vi "Amira Bladder Calibration.vi"() -> ()   [LabVIEW 2020]
uses:
  <userlib>/KQD LabVIEW User/Serial/Controls/SERIAL PortConfig.ctl
  <userlib>/KQD LabVIEW User/Serial/Controls/SERIAL BaudRate.ctl
  <userlib>/Amira UART/Public/TypeDefs/AUART StepDir.ctl
  <userlib>/Amira UART/Amira UART.lvclass
  <userlib>/KQD LabVIEW User/Serial/Serial.lvlib
panel:
  in  "RunWith":cluster{"Steps":i32, "Rates":i32}={"Steps"=400, "Rates"=40}
  in  "Folder":path=path "C:/Amira Data/Strip"
  in  "Strip":enum16{"Surface", "Blader"}(ring)
  out "FrontOpen":dbl
  out "BackOpen":dbl
  out "FrontClose":dbl
  out "BackClose":dbl
  in  "StartAt":cluster{"Steps":i32, "Rates":i32}={"Steps"=950, "Rates"=200}
  out "Position":dbl[](graph)
  in  "DAQ":tag="Dev1/port0"
  out "UART":string
  in  "ComPort":refnum<visa-resource-name>
  in  "Config":T1={"BaudRate"=enum."460800", "StopBits"=10, "DataBits"=8, "Parity"=enum."None", "FlowControl"=2, "TimeOut"=1000, "TermChar"=10, "ReadTermEn"=TRUE} {"TermChar" format="%.0x"; "FlowControl" items=["None", "XON/XOFF", "RTS/CTS", "XON/XOFF & RTS/CTS", "DTR/DSR", "XON/XOFF & DTR/DSR"]; "DataBits" min=5 max=8 step=1; "StopBits" items=["1.0"=10, "1.5"=15, "2.0"=20]}
  out "ErrOut":errorcluster
  in  "ErrIn":errorcluster
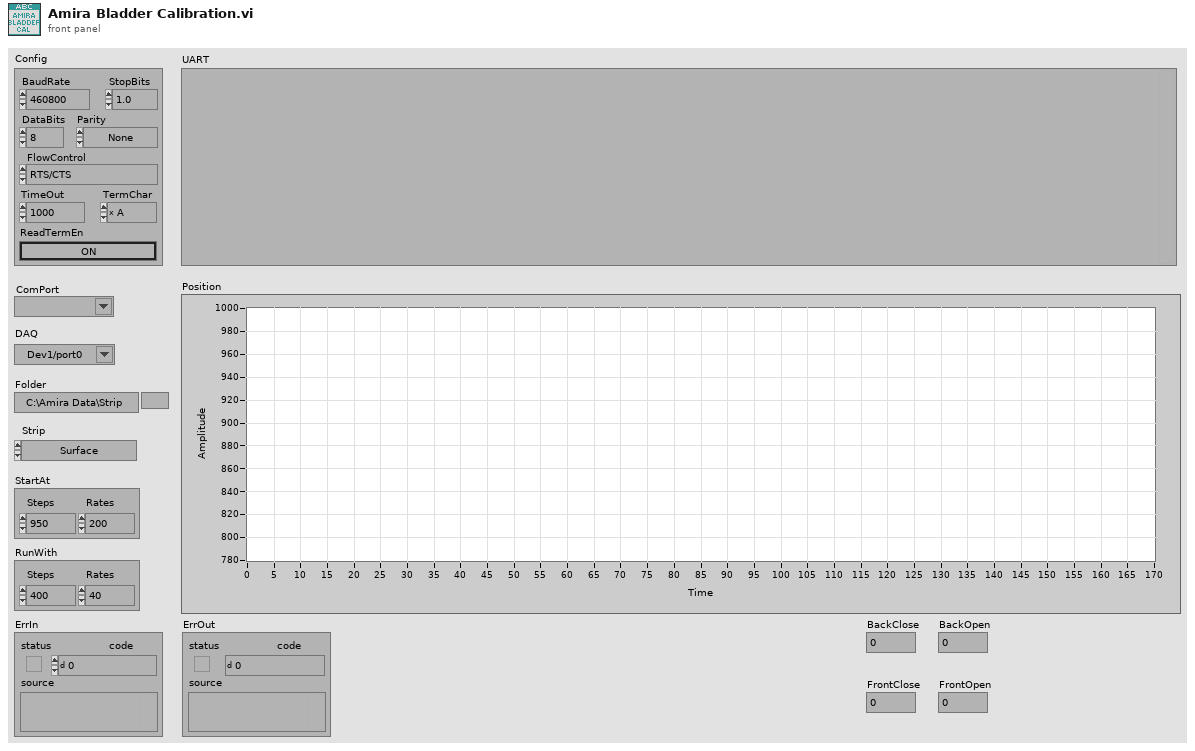
[diagram p1: front panel]
types:
  T1 = typedef "Serial.lvlib/SERIAL PortConfig.ctl" = cluster{"BaudRate":T2, "StopBits":u16, "DataBits":u16, "Parity":enum16{"None", "Odd", "Even", "Mark", "Space"}, "FlowControl":u16, "TimeOut":u32, "TermChar":u8, "ReadTermEn":bool}
  T2 = typedef "SERIAL BaudRate.ctl" = enum16{"2400", "4800", "7200", "9600", "14400", "19200", "28800", "38400", "57600", "115200", "128000", "230400", "460800", "921600"}
  T3 = typedef "Amira UART.lvclass/AUART StepDir.ctl" = enum16{"", "compress", "decompress"}
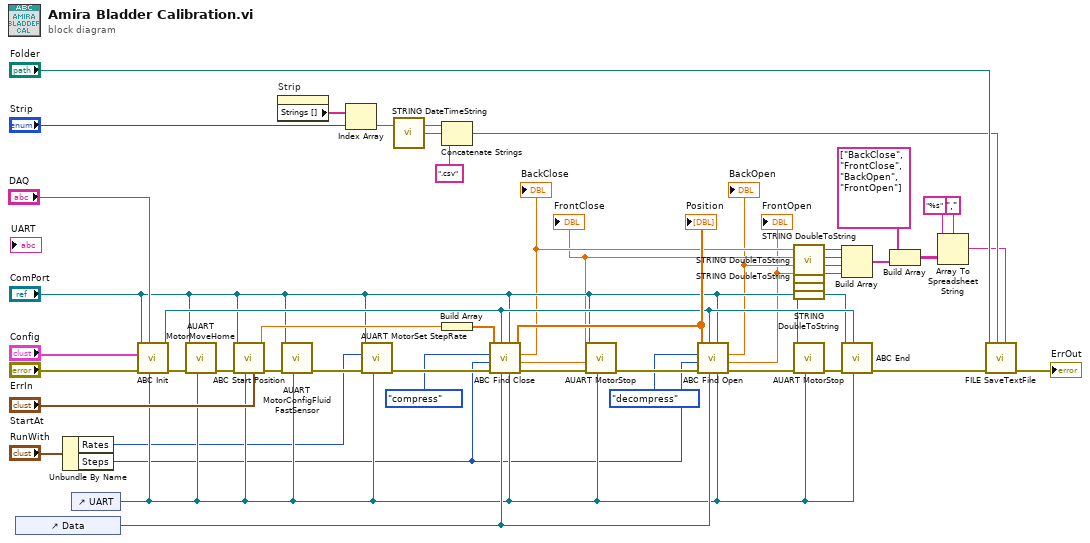
[diagram p0: block diagram]
diagram:
  n1 = control-ref of="Data"() -> (w32:refnum<vi>)
  n2 = Unbundle By Name("RunWith") -> ("Rates"=w2:i32, "Steps"=w1:i32)
  n3 = control-ref of="UART"() -> (w29:refnum<vi>)
  n4 = call "ABC Init.vi"("UART"=w29, "DAQ"="DAQ", "ErrIn"="ErrIn", "PortConfig"="Config", "ComPort"="ComPort") -> ("ErrOut"=w44:errorcluster, "DaqTask"=w33:refnum<k21>)  [unwired: 5 in]
  n5 = call <userlib>:"AUART MotorMoveHome.vi"("UART"=w29, "ErrIn"=w44, "Port"="ComPort") -> ("ErrOut"=w43:errorcluster)  [unwired: 7 in, 1 out]
  n6 = call "ABC Start Position.vi"("Start"="StartAt", "UART"=w29, "ErrIn"=w43, "ComPort"="ComPort") -> ("ErrOut"=w42:errorcluster, "LastPos"=w39:dbl)  [unwired: 6 in]
  n7 = property on="Strip" class="Enum (strict)"() -> ("Strings []"=w22:string[])  [unwired: 2 in, 2 out]
  n8 = call <userlib>:"AUART MotorConfigFluidFastSensor.vi"("UART"=w29, "ErrIn"=w42, "Port"="ComPort") -> ("ErrOut"=w46:errorcluster)  [unwired: 8 in]
  n9 = Index Array(array=w22, index="Strip") -> (element=w20:string)
  n10 = call <userlib>:"AUART MotorSet StepRate.vi"("UART"=w29, "ErrIn"=w46, "step_rate"=w2, "Port"="ComPort") -> ("ErrOut"=w45:errorcluster)  [unwired: 7 in]
  n11 = call <userlib>:"STRING DateTimeString.vi"() -> ("DateTimeStr"=w19:string)  [unwired: 2 in]
  n12 = Concatenate Strings(w20, w19, ".csv" ("string")) -> (w16:string)
  n13 = Build Array(w39) -> (w40:dbl[])
  n14 = call "ABC Find Close.vi"("UART"=w29, "ComPort"="ComPort", "Data"=w32, "DaqTask"=w33, "ErrIn"=w45, "#Step"=w1, "Dir"=AUART_StepDir."compress" ("step_dir"), "DataIn"=w40) -> ("ErrOut"=w37:errorcluster, "FrontClose"=w27:dbl, "BackClose"=w28:dbl, "DataOut"=w34:dbl[])
  "Position" <- w34
  "BackClose" <- w28
  "FrontClose" <- w27
  n15 = call <userlib>:"AUART MotorStop.vi"("UART"=w29, "ErrIn"=w37, "Port"="ComPort") -> ("ErrOut"=w36:errorcluster)  [unwired: 8 in]
  n16 = call "ABC Find Open.vi"("UART"=w29, "ComPort"="ComPort", "Data"=w32, "DaqTask"=w33, "ErrIn"=w36, "#Step"=w1, "Dir"=AUART_StepDir."decompress" ("step_dir"), "DataIn"=w34) -> ("ErrOut"=w35:errorcluster, "FrontOpen"=w25:dbl, "BackOpen"=w26:dbl)  [unwired: 1 out]
  "BackOpen" <- w26
  "FrontOpen" <- w25
  n17 = call <userlib>:"STRING DoubleToString.vi"("Num"=w28) -> ("DblStr"=w15:string)  [unwired: 3 in]
  n18 = call <userlib>:"STRING DoubleToString.vi"("Num"=w27) -> ("DblStr"=w14:string)  [unwired: 3 in]
  n19 = call <userlib>:"STRING DoubleToString.vi"("Num"=w26) -> ("DblStr"=w13:string)  [unwired: 3 in]
  n20 = call <userlib>:"STRING DoubleToString.vi"("Num"=w25) -> ("DblStr"=w12:string)  [unwired: 3 in]
  n21 = call <userlib>:"AUART MotorStop.vi"("UART"=w29, "ErrIn"=w35, "Port"="ComPort") -> ("ErrOut"=w30:errorcluster)  [unwired: 8 in]
  n22 = Build Array(w15, w14, w13, w12) -> (w10:string[])
  n23 = call "ABC End.vi"("UART"=w29, "DaqTask"=w33, "ErrIn"=w30, "ComPort"="ComPort") -> ("ErrOut"=w24:errorcluster)  [unwired: 7 in]
  n24 = Build Array(string[] ["BackClose", "FrontClose", "BackOpen", "FrontOpen"], w10) -> (w9:string[][])
  n25 = Array To Spreadsheet String(delimiter (Tab)=",", array=w9, 3:"%s" ("format string")) -> (spreadsheet string=w7:string)
  n26 = call <userlib>:"FILE SaveTextFile.vi"("Data"=w7, "File"=w16, "ErrIn"=w24, "Folder"="Folder") -> ("ErrOut"=→"ErrOut":errorcluster)  [unwired: 7 in]
